vi "gl_8-bit montage window ctrl refs.vi"() -> ()   [LabVIEW 2013]
uses:
  Timelapse Viewer/Typedefs/8-bit video export window ctrl refs.ctl
  Typedefs/Bright-Contr-Gamma cluster.ctl
  Timelapse Viewer/Typedefs/Speed graph behaviour enum.ctl
panel:
  in  "Output video file path":path
  in  "8-bit montage window ctrl refs":T1
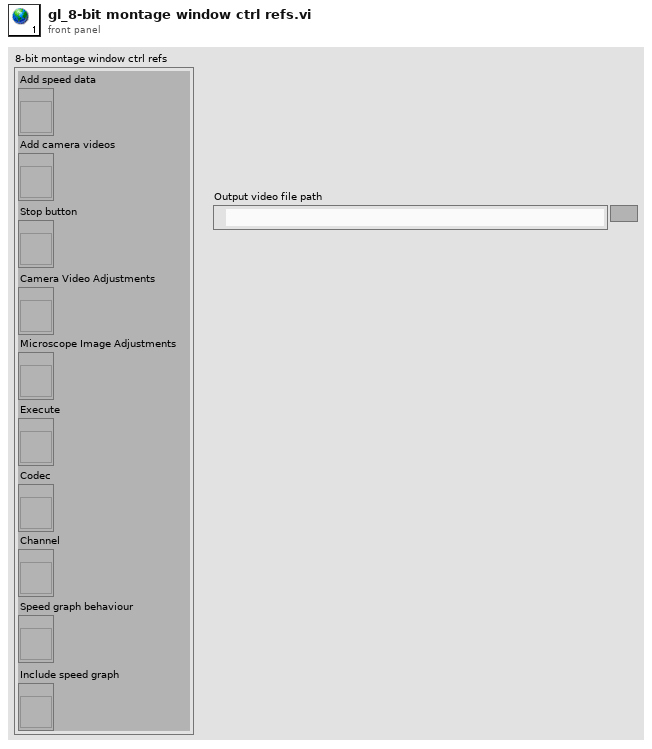
[diagram p1: front panel]
types:
  T1 = typedef "8-bit video export window ctrl refs.ctl" = cluster{"Add speed data":refnum<vi>, "Add camera videos":refnum<vi>, "Stop button":refnum<vi>, "Camera Video Adjustments":refnum<vi>, "Microscope Image Adjustments":refnum<vi>, "Execute":refnum<vi>, "Codec":refnum<vi>, "Channel":refnum<vi>, "Speed graph behaviour":refnum<vi>, "Include speed graph":refnum<vi>}
diagram:
